vi "Convert CBOR Hex Integer.vi"(2 "Structure":u8, 3 "CBOR Hex":string) -> (0 "{Integer}":string)   [LabVIEW 2020, in "CBOR.lvlib"]
doc: "Convert CBOR HEX into Integer."
uses:
  CBOR.lvlib
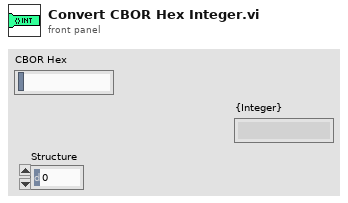
[diagram p1: front panel]
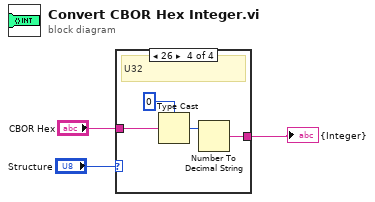
[diagram p0: block diagram]
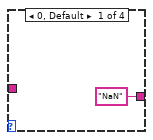
[diagram p2: hidden frame]
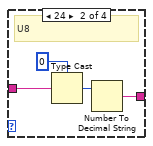
[diagram p3: hidden frame]
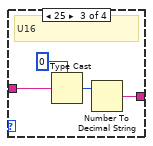
[diagram p4: hidden frame]
diagram:
  n1 = case shown="26" "Structure" {
    tunnel: "CBOR Hex" -> [_ w8 w12 w16]
    tunnel: ["NaN" w5 w9 w13] -> w1
    frame 0, Default {
    }
    frame 24 {
      # "U8"
      n2 = Type Cast(type=u8 0, x=w8) -> (*(type *) &x=w6:u8)
      n3 = Number To Decimal String(number=w6) -> (decimal integer string=w5:string)  [unwired: 1 in]
    }
    frame 25 {
      # "U16"
      n4 = Type Cast(type=u16 0, x=w12) -> (*(type *) &x=w10:u16)
      n5 = Number To Decimal String(number=w10) -> (decimal integer string=w9:string)  [unwired: 1 in]
    }
    frame 26 {
      # "U32"
      n6 = Type Cast(type=u32 0, x=w16) -> (*(type *) &x=w14:u32)
      n7 = Number To Decimal String(number=w14) -> (decimal integer string=w13:string)  [unwired: 1 in]
    }
  }
  "{Integer}" <- w1
